vi "FT10_Read LVM File.vi"() -> ()   [LabVIEW 2024]
uses:
  <vilib>/Waveform/WDTOps.llb/WDT Waveform Duration DBL.vi
panel:
  in  "path to JPEG file":path
  in  "path to PNG file":path
  in  "Save Graph":bool
  out "Y min":dbl format="%0.2f"
  out "Y max":dbl format="%0.2f"
  out "X Max":dbl format="%0.6f"
  in  "Y Scale.Range:Maximum":dbl
  in  "Y Scale.Range:Minimum":dbl
  in  "X Scale.Range:Maximum":dbl=0.0015
  in  "X Scale.Range:Minimum":dbl
  in  "stop":bool
  out "Waveform Graph":dynamicdata(graph)
  in  "Filename":path=path "C:/Users/yearon2/OneDrive - Medtronic PLC/LV2015/LT10 Generator Sandbox/FT10_rev2/Data"
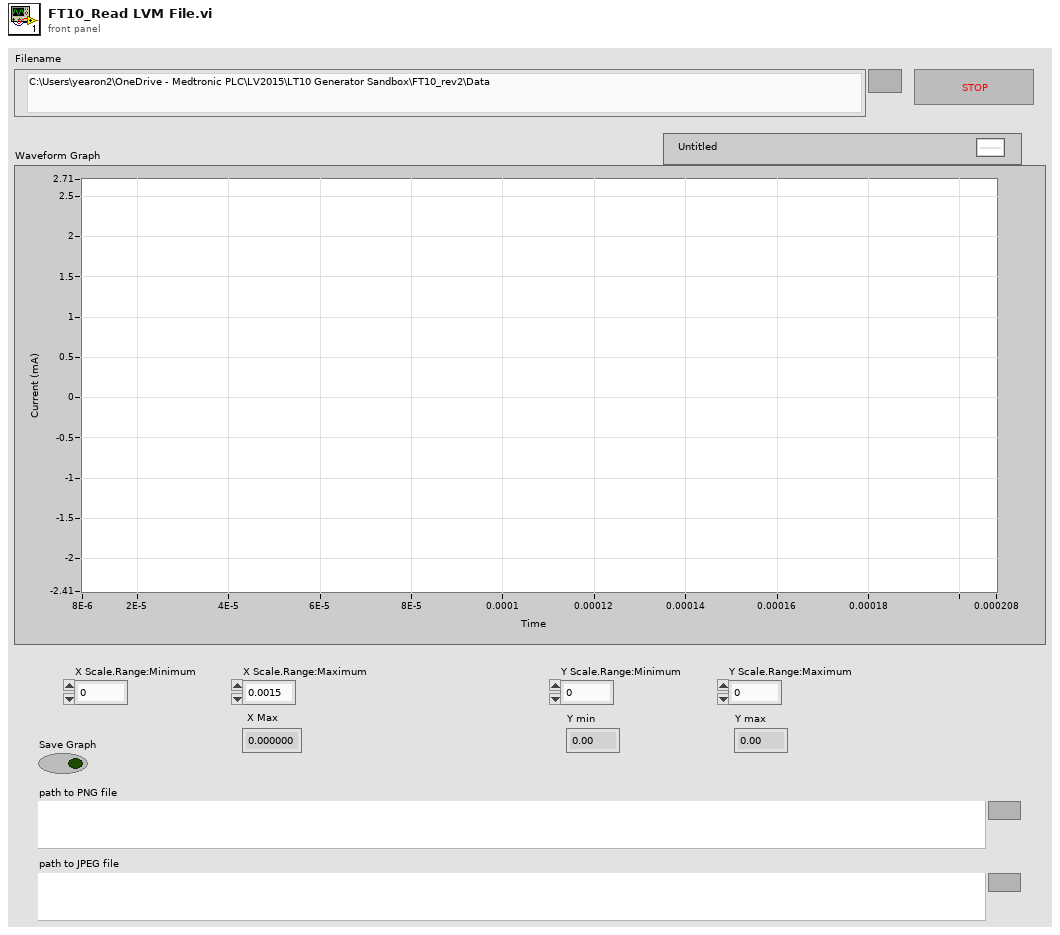
[diagram p1: front panel]
types:
  T1 = typedef "imagedata.ctl" = cluster{"image type":i32, "image depth":i32, "image":u8[], "mask":u8[], "colors":u32[], "Rectangle":cluster{"left":i16, "top":i16, "right":i16, "bottom":i16}}
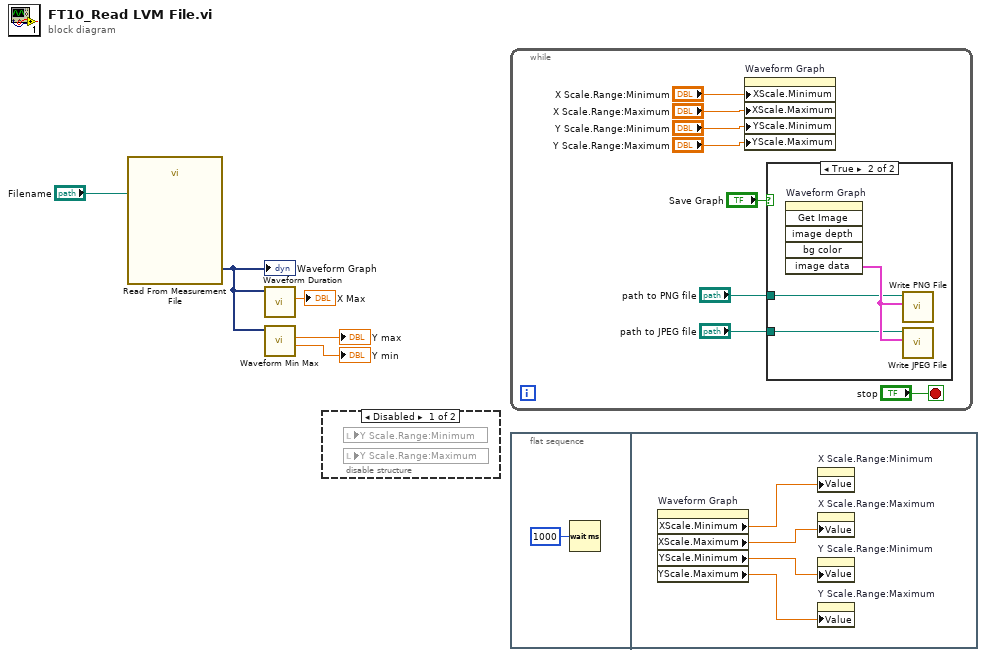
[diagram p0: block diagram]
diagram:
  n1 = call "Read From Measurement File"("Filename"="Filename") -> ("Signals"=w4:dynamicdata)  [unwired: 5 in, 5 out]
  "Waveform Graph" <- w4
  n2 = call-poly <vilib>:"Waveform Duration.vi"("waveform in"=w4) -> ("duration"=→"X Max":dbl)  [unwired: 8 in, 2 out]
  n3 = call <vilib>:"Waveform Min Max.vi"("waveform in"=w4) -> ("Y min"=→"Y min":dbl, "Y max"=→"Y max":dbl)  [unwired: 5 in, 4 out]
  n4 = disable-structure shown="Disabled" {
    frame Disabled {
      n5 = local read "Y Scale.Range:Minimum"() -> ()  [unwired: 1 in]
      n6 = local read "Y Scale.Range:Maximum"() -> ()  [unwired: 1 in]
    }
    frame Enabled {
    }
  }
  n7 = while {
    stop <- "stop" stop-if-true
    n8 = property on="Waveform Graph" class="WFGraph (strict)"("XScale.Minimum"="X Scale.Range:Minimum", "XScale.Maximum"="X Scale.Range:Maximum", "YScale.Minimum"="Y Scale.Range:Minimum", "YScale.Maximum"="Y Scale.Range:Maximum") -> ()  [unwired: 2 in, 2 out]
    n9 = case shown="True" "Save Graph" {
      tunnel: "path to PNG file" -> [_ w15]
      tunnel: "path to JPEG file" -> [_ w14]
      frame False {
      }
      frame True {
        n10 = invoke on="Waveform Graph" class="WFGraph (strict)" method="Get Image"() -> ("image data"=w16:T1)  [unwired: 6 in, 5 out]
        n11 = call <vilib>:"Write PNG File.vi"("image data"=w16, "path to PNG file"=w15) -> ()  [unwired: 8 in, 2 out]
        n12 = call <vilib>:"Write JPEG File.vi"("image data"=w16, "path to JPEG file"=w14) -> ()  [unwired: 8 in, 2 out]
      }
    }
  }
  n13 = flat-sequence {
    frame #0 {
      n14 = Wait (ms)(milliseconds to wait=u32 1000) -> ()  [unwired: 1 out]
    }
    frame #1 {
      n15 = property on="Waveform Graph" class="WFGraph (strict)"() -> ("XScale.Minimum"=w21:dbl, "XScale.Maximum"=w20:dbl, "YScale.Minimum"=w19:dbl, "YScale.Maximum"=w18:dbl)  [unwired: 2 in, 2 out]
      n16 = property on="X Scale.Range:Minimum" class="DigNum (strict)"("Value"=w21) -> ()  [unwired: 2 in, 2 out]
      n17 = property on="X Scale.Range:Maximum" class="DigNum (strict)"("Value"=w20) -> ()  [unwired: 2 in, 2 out]
      n18 = property on="Y Scale.Range:Minimum" class="DigNum (strict)"("Value"=w19) -> ()  [unwired: 2 in, 2 out]
      n19 = property on="Y Scale.Range:Maximum" class="DigNum (strict)"("Value"=w18) -> ()  [unwired: 2 in, 2 out]
    }
  }
